vi "Init.vi"(4 "Message Cfg":T1={"EnTermChar"=TRUE, "termChar"=13, "suppEnEnRd"=FALSE, "sendEndEn"=TRUE} {"termChar" format="%.0x"}, 6 "timeout":u32=1000, 7 "Name":string, 8 "error in":errorcluster, 9 "serialCfg":T2={"baud rate (9600)"=19200, "data bits (8)"=8, "stop bits (10: 1 bit)"=10, "parity (0:none)"=enum."None", "flow control (0:none)"=0, "endModeforReads"=0, "endModeforWrites"=0} {"endModeforWrites" items=["None", "Last Bit", "TermChar", "Break"]; "endModeforReads" items=["None", "Last Bit", "TermChar"]; "flow control (0:none)" items=["None", "XON/XOFF", "RTS/CTS", "XON/XOFF & RTS/CTS", "DTR/DSR", "XON/XOFF & DTR/DSR"]; "stop bits (10: 1 bit)" items=["1.0"=10, "1.5"=15, "2.0"=20]; "data bits (8)" min=5 max=8 step=1}, 10 "Port":refnum<visa-resource-name>, 11 "Vaisala Probe in":refnum<class "Vaisala Probe.lvclass">) -> (0 "error out":errorcluster, 3 "Vaisala Probe out":refnum<class "Vaisala Probe.lvclass">)   [LabVIEW 2013, in "Vaisala Probe.lvclass"]
doc: "Initialize communication with a serial port. Open the port and obtain a reference to a semaphore that will be used to prevent communication clashes. If the device is recorded as \"present\" at initialization, then the port will be closed and initialization will then proceed as intended."
uses:
  Vaisala Probe.lvclass
  Reusable/Serial IO/Serial IO.lvclass
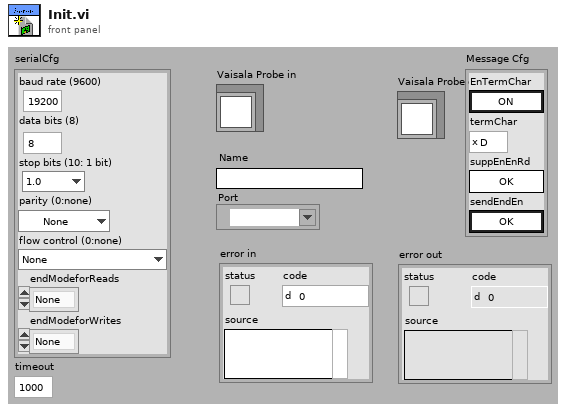
[diagram p1: front panel]
types:
  T1 = cluster{"EnTermChar":bool, "termChar":u8, "suppEnEnRd":bool, "sendEndEn":bool}
  T2 = cluster{"baud rate (9600)":u32, "data bits (8)":u16, "stop bits (10: 1 bit)":u16, "parity (0:none)":enum16{"None", "Odd", "Even", "Mark", "Space"}, "flow control (0:none)":u16, "endModeforReads":u16, "endModeforWrites":u16}
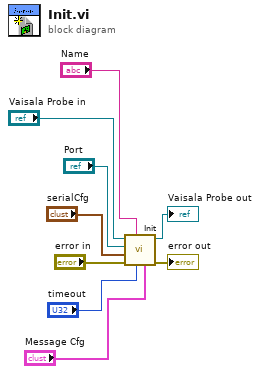
[diagram p0: block diagram]
diagram:
  n1 = call-parent "Init.vi"("Message Cfg"="Message Cfg", "timeout"="timeout", "Name"="Name", "error in"="error in", "serialCfg"="serialCfg", "Port"="Port", "Serial IO in"="Vaisala Probe in") -> ("error out"=→"error out":errorcluster, "Serial IO out"=→"Vaisala Probe out":refnum<class "Vaisala Probe.lvclass">)  [unwired: 3 in]
